vi "Stage group check.vi"(8 "error in (no error)":errorcluster, 9 "XPS error in (no error)":errorcluster, 10 "Group Name (250 c max)":string, 11 "connection ID in":T1) -> (0 "error out":errorcluster, 1 "XPS error out":errorcluster, 2 "Stages ready?":bool, 3 "connection ID out":T1, 5 "Group Name (250 c max) 2":string)   [LabVIEW 2016]
panel:
  in  "Status codes":i32[](array[numeric])=[10, 11, 12, 13, 14, 15, 16, 17, 18]
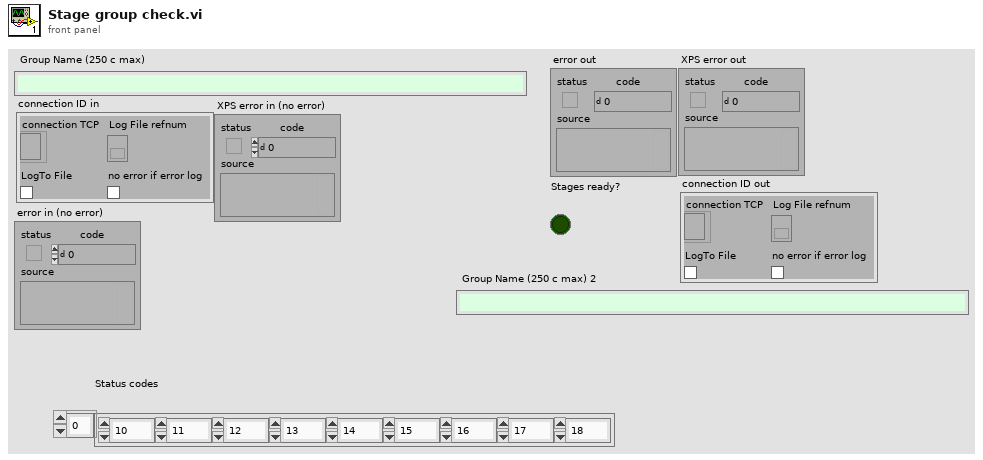
[diagram p1: front panel]
types:
  T1 = cluster{"connection TCP":refnum<k5>, "LogTo File":bool, "Log File refnum":refnum<file>, "no error if error log":bool}
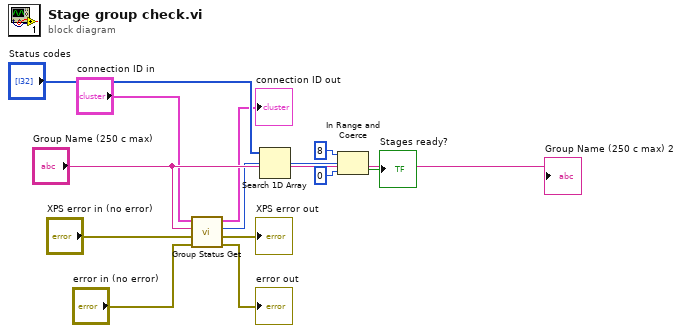
[diagram p0: block diagram]
diagram:
  n1 = call <userlib>:"Group Status Get.vi"("error in (no error)"="error in (no error)", "XPS error in (no error)"="XPS error in (no error)", "Group Name (250 c max)"="Group Name (250 c max)", "connection ID in"="connection ID in") -> ("error out"=→"error out":errorcluster, "XPS error out"=→"XPS error out":errorcluster, "Status"=w6:i32, "connection ID out"=→"connection ID out":T1)  [unwired: 4 in]
  n2 = Search 1D Array(1D array="Status codes", element=w6) -> (index of element=w4:i32)  [unwired: 1 in]
  n3 = In Range and Coerce(upper limit=8, x=w4, lower limit=0) -> (In Range?=→"Stages ready?":bool)  [unwired: 1 out]
  "Group Name (250 c max) 2" <- "Group Name (250 c max)"
